vi "Encode Payload Data from Channels.vi"(6 "Offset":i32, 8 "error in":errorcluster, 9 "Parameters":T2(array[cluster]) {"encoding" items=["BNR", "BCD", "Discrete", "Signed_32", "Signed_64", "Float_32", "Float_64", "Opaque"]}, 10 "Data in":u8[](array[numeric]), 11 "Values in":dbl[](array[numeric])) -> (0 "error out":errorcluster, 2 "Data out":u8[](array[numeric]), 4 "Number of Parameters":i32)   [LabVIEW 2020]
uses:
  Encoding (Arinc664).ctl
  b24d3698-aaae-4200-bf93-4b6af5480478.vi
  5b1080be-549e-4688-aad8-fb955257d8ef.vi
  2afa5e5b-ae47-4ac6-b34f-e51087edfaba.vi
  1eaed3cb-9180-4944-bca4-c812fd7aad88.vi
  f46899e6-f3c2-4da0-acc2-ed34a334556c.vi
  7b487445-4b60-493e-9c15-0f5b7677c2b1.vi
  7e7e8f0d-6015-4215-b4f4-37ecf7ce16f3.vi
  b24d3698-aaae-4200-bf93-4b6af5480478.vi/9377bb8f-44b5-4a8f-87f1-966fd5a9edcc.vi
  b24d3698-aaae-4200-bf93-4b6af5480478.vi/e95d9d1f-307c-44d6-9f26-c3f519a4990d.vi
  b24d3698-aaae-4200-bf93-4b6af5480478.vi/0c23f515-4369-4514-bc3d-4444e6b437b2.vi
  5b1080be-549e-4688-aad8-fb955257d8ef.vi/136dcdcb-2dd3-4a4d-a796-a8f7a3f8e1ac.vi
  5b1080be-549e-4688-aad8-fb955257d8ef.vi/a54b505c-1216-4ef4-8378-3ceda9d188df.vi
  <vilib>/NI/NI VeriStand Encoding and Decoding/Get Bits Per Digit from Base.vi
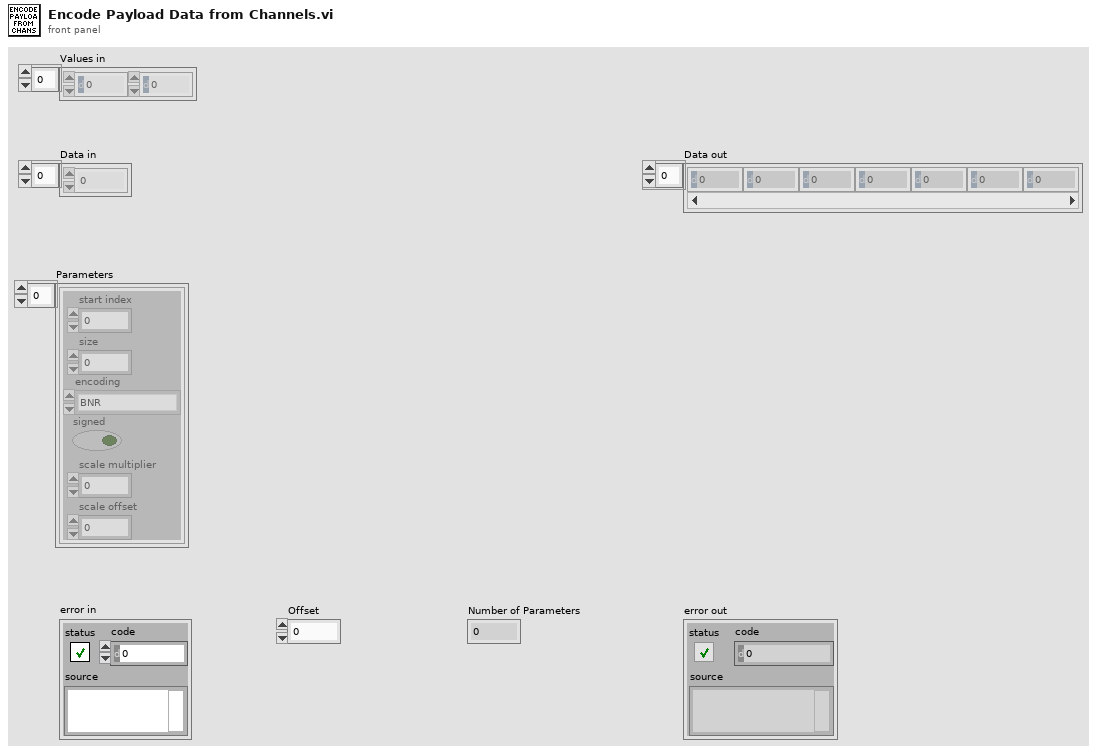
[diagram p1: front panel]
types:
  T1 = typedef "Encoding (Arinc664).ctl" = u16
  T2 = cluster{"start index":i32, "size":i32, "encoding":T1, "signed":bool, "scale multiplier":dbl, "scale offset":dbl}[]
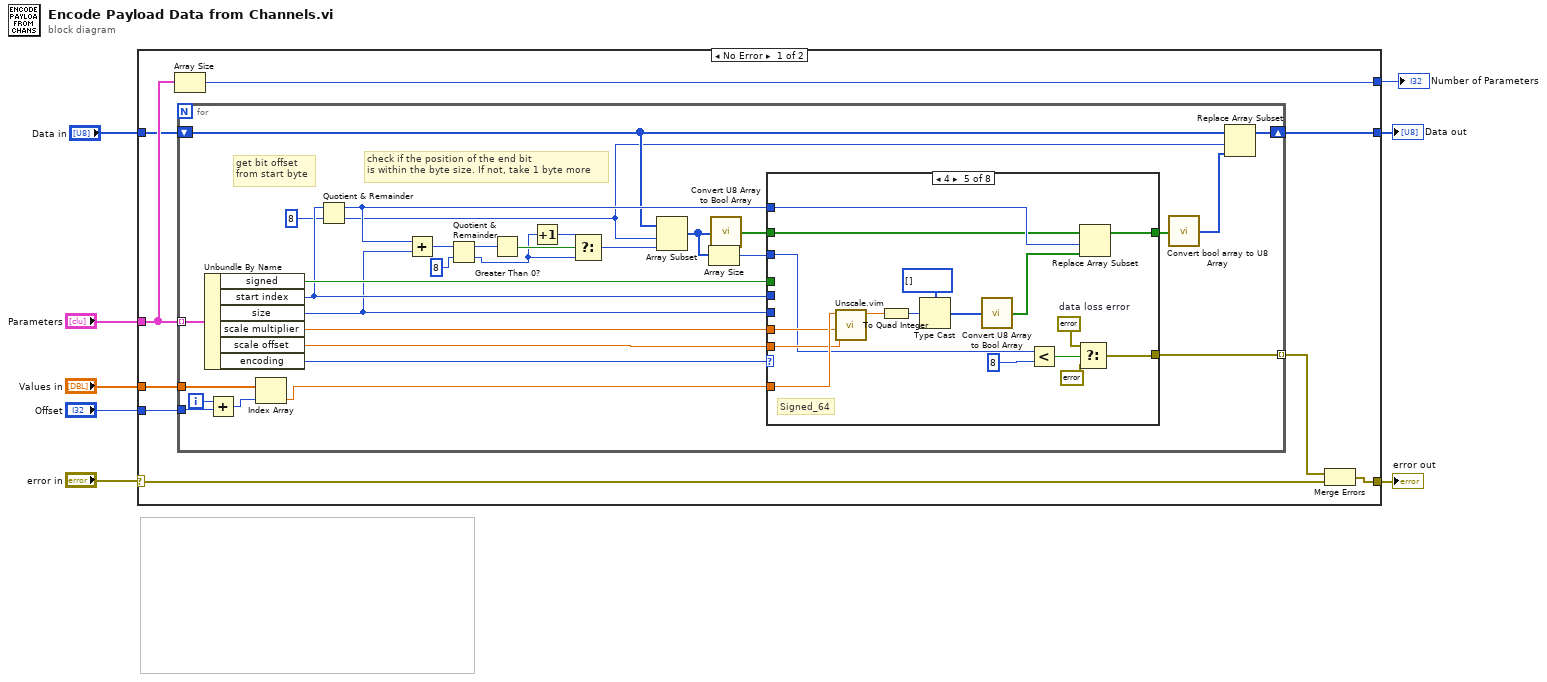
[diagram p0: block diagram]
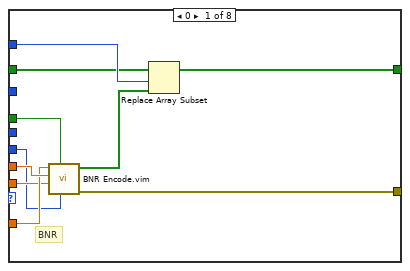
[diagram p2: hidden frame]
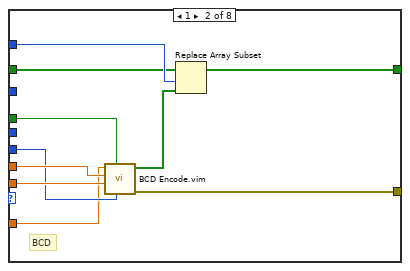
[diagram p3: hidden frame]
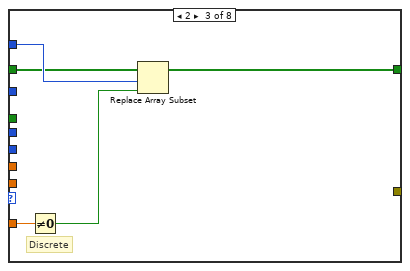
[diagram p4: hidden frame]
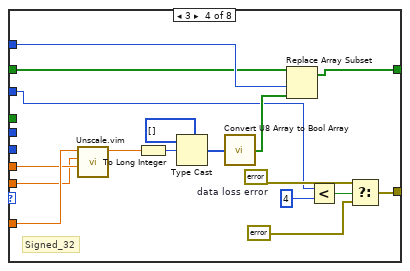
[diagram p5: hidden frame]
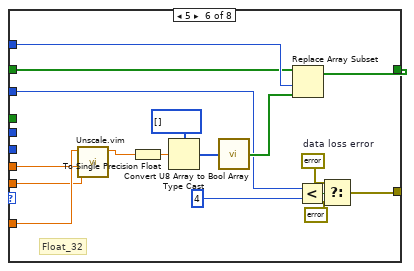
[diagram p6: hidden frame]
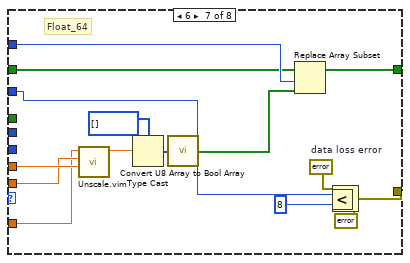
[diagram p7: hidden frame]
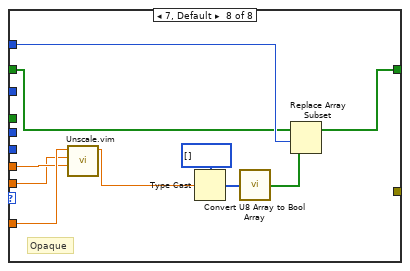
[diagram p8: hidden frame]
diagram:
  n1 = case shown="No Error" "error in" {
    selector: "error in" -> [w13 w151]
    tunnel: "Values in" -> [w17 _]
    tunnel: [w16 w150] -> w7
    tunnel: [w14 w151] -> w5
    tunnel: "Offset" -> [w12 _]
    tunnel: [w11 _] -> w3
    tunnel: "Parameters" -> [w10 _]
    tunnel: "Data in" -> [w9 w150]
    frame No Error {
      n2 = Array Size(array=w10) -> (size(s)=w11:i32)
      n3 = for {
        tunnel: w17 -> [w46]
        tunnel: w10 -> [w47] mode=indexing
        shift-right: [w24] -> w16
        shift-left: w9 -> [w25]
        tunnel: [w45] -> w15 mode=indexing
        tunnel: w12 -> [w43]
        i -> [w44]
        # "check if the position of the end bit \nis within the byte size. If not, take 1 byte more"
        # "get bit offset\nfrom start byte"
        n4 = Unbundle By Name(w47) -> ("signed"=w37:bool, "start index"=w36:i32, "size"=w33:i32, "scale multiplier"=w39:dbl, "scale offset"=w38:dbl, "encoding"=w40:T1)
        n5 = Add(x=w44, y=w43) -> (x+y=w42:i32)
        n6 = Index Array(array=w46, index=w42) -> (element=w41:dbl)
        n7 = Quotient & Remainder(x=w36, y=8) -> (x-y*floor(x/y)=w34:i32, floor(x/y)=w21:i32)
        n8 = Add(x=w34, y=w33) -> (x+y=w32:i32)
        n9 = Quotient & Remainder(x=w32, y=8) -> (x-y*floor(x/y)=w30:i32, floor(x/y)=w28:i32)
        n10 = Greater Than 0?(x=w30) -> (x > 0?=w29:bool)
        n11 = Increment(x=w28) -> (x+1=w27:i32)
        n12 = Select(t=w27, s=w29, f=w28) -> (s? t:f=w20:i32)
        n13 = Array Subset(array=w25, index=w21, length=w20) -> (w18:u8[])
        n14 = Array Size(array=w18) -> (size(s)=w19:i32)
        n15 = call "Convert U8 Array to Bool Array.vi"("U8 array in"=w18) -> ("Boolean array out"=w26:bool[])  [unwired: 14 in]
        n16 = case shown="4" w40 {
          tunnel: w37 -> [w57 w67 _ _ _ _ _ _]
          tunnel: w39 -> [w56 w66 _ w87 w104 w121 w138 w147]
          tunnel: w38 -> [w54 w65 _ w86 w103 w120 w137 w146]
          tunnel: w36 -> [_ _ _ _ _ _ _ _]
          tunnel: w33 -> [w53 w64 _ _ _ _ _ _]
          tunnel: w41 -> [w55 w62 w71 w88 w105 w122 w128 w148]
          tunnel: w34 -> [w52 w60 w72 w89 w106 w123 w139 w149]
          tunnel: [w50 w63 _ w80 w97 w114 w132 _] -> w45
          tunnel: w26 -> [w49 w59 w69 w75 w91 w108 w126 w141]
          tunnel: [w48 w58 w68 w74 w92 w109 w124 w140] -> w23
          tunnel: w19 -> [_ _ _ w73 w90 w107 w125 _]
          frame 0 {
            # "BNR"
            n17 = call "BNR Encode.vim"("data size (bits)"=w53, "signed"=w57, "scale offset"=w54, "scale multiplier"=w56, "value"=w55) -> ("error out"=w50:errorcluster, "BNR encoded value"=w51:bool[])  [unwired: 5 in]
            n18 = Replace Array Subset(array=w49, new element=w51, index=w52) -> (w48:bool[])
          }
          frame 1 {
            # "BCD"
            n19 = call "BCD Encode.vim"("data size (bits)"=w64, "signed"=w67, "scale offset"=w65, "scale multiplier"=w66, "value"=w62) -> ("error out"=w63:errorcluster, "BCD encoded value"=w61:bool[])  [unwired: 4 in, 1 out]
            n20 = Replace Array Subset(array=w59, new element=w61, index=w60) -> (w58:bool[])
          }
          frame 2 {
            # "Discrete"
            n21 = Not Equal To 0?(x=w71) -> (x != 0?=w70:bool)
            n22 = Replace Array Subset(array=w69, new element=w70, index=w72) -> (w68:bool[])
          }
          frame 3 {
            w81 = errorcluster {"status"=TRUE, "code"=-732301, "source"="data loss during encoding"}  # data loss error
            # "Signed_32"
            n23 = call "Unscale.vim"("scale multiplier"=w87, "scale offset"=w86, "value"=w88) -> ("unscaled value"=w85:dbl)  [unwired: 8 in]
            n24 = To Long Integer(number=w85) -> (32bit integer=w76:i32)
            n25 = Type Cast(type=u8[] [] ("subarray"), x=w76) -> (*(type *) &x=w83:u8[])
            n26 = call "Convert U8 Array to Bool Array.vi"("U8 array in"=w83) -> ("Boolean array out"=w82:bool[])  [unwired: 14 in]
            n27 = Replace Array Subset(array=w75, new element=w82, index=w89) -> (w74:bool[])
            n28 = Less?(x=w73, y=4) -> (x < y?=w78:bool)
            n29 = Select(t=w81, s=w78, f=errorcluster {"status"=FALSE, "code"=0, "source"=""}) -> (s? t:f=w80:errorcluster)
          }
          frame 4 {
            w98 = errorcluster {"status"=TRUE, "code"=-732301, "source"="data loss during encoding"}  # data loss error
            # "Signed_64"
            n30 = call "Unscale.vim"("scale multiplier"=w104, "scale offset"=w103, "value"=w105) -> ("unscaled value"=w102:dbl)  [unwired: 8 in]
            n31 = To Quad Integer(1:w102) -> (0:w93:i64)
            n32 = Type Cast(type=u8[] [] ("subarray"), x=w93) -> (*(type *) &x=w100:u8[])
            n33 = call "Convert U8 Array to Bool Array.vi"("U8 array in"=w100) -> ("Boolean array out"=w99:bool[])  [unwired: 14 in]
            n34 = Less?(x=w90, y=8) -> (x < y?=w95:bool)
            n35 = Select(t=w98, s=w95, f=errorcluster {"status"=FALSE, "code"=0, "source"=""}) -> (s? t:f=w97:errorcluster)
            n36 = Replace Array Subset(array=w91, new element=w99, index=w106) -> (w92:bool[])
          }
          frame 5 {
            w115 = errorcluster {"status"=TRUE, "code"=-732301, "source"="data loss during encoding"}  # data loss error
            # "Float_32"
            n37 = call "Unscale.vim"("scale multiplier"=w121, "scale offset"=w120, "value"=w122) -> ("unscaled value"=w119:dbl)  [unwired: 8 in]
            n38 = To Single Precision Float(number=w119) -> (single precision float=w110:sgl)
            n39 = Type Cast(type=u8[] [] ("subarray"), x=w110) -> (*(type *) &x=w117:u8[])
            n40 = call "Convert U8 Array to Bool Array.vi"("U8 array in"=w117) -> ("Boolean array out"=w116:bool[])  [unwired: 14 in]
            n41 = Replace Array Subset(array=w108, new element=w116, index=w123) -> (w109:bool[])
            n42 = Less?(x=w107, y=4) -> (x < y?=w112:bool)
            n43 = Select(t=w115, s=w112, f=errorcluster {"status"=FALSE, "code"=0, "source"=""}) -> (s? t:f=w114:errorcluster)
          }
          frame 6 {
            w133 = errorcluster {"status"=TRUE, "code"=-732301, "source"="data loss during encoding"}  # data loss error
            # "Float_64"
            n44 = call "Unscale.vim"("scale multiplier"=w138, "scale offset"=w137, "value"=w128) -> ("unscaled value"=w127:dbl)  [unwired: 8 in]
            n45 = Type Cast(type=u8[] [] ("subarray"), x=w127) -> (*(type *) &x=w135:u8[])
            n46 = call "Convert U8 Array to Bool Array.vi"("U8 array in"=w135) -> ("Boolean array out"=w134:bool[])  [unwired: 14 in]
            n47 = Replace Array Subset(array=w126, new element=w134, index=w139) -> (w124:bool[])
            n48 = Less?(x=w125, y=8) -> (x < y?=w130:bool)
            n49 = Select(t=w133, s=w130, f=errorcluster {"status"=FALSE, "code"=0, "source"=""}) -> (s? t:f=w132:errorcluster)
          }
          frame 7, Default {
            # "Opaque"
            n50 = call "Unscale.vim"("scale multiplier"=w147, "scale offset"=w146, "value"=w148) -> ("unscaled value"=w145:dbl)  [unwired: 8 in]
            n51 = Type Cast(type=u8[] [] ("subarray"), x=w145) -> (*(type *) &x=w143:u8[])
            n52 = call "Convert U8 Array to Bool Array.vi"("U8 array in"=w143) -> ("Boolean array out"=w142:bool[])  [unwired: 14 in]
            n53 = Replace Array Subset(array=w141, new element=w142, index=w149) -> (w140:bool[])
          }
        }
        n54 = call "Convert bool array to U8 Array.vi"("Boolean array"=w23) -> ("Array"=w22:u8[])  [unwired: 14 in]
        n55 = Replace Array Subset(array=w25, new element=w22, index=w21) -> (w24:u8[])
      }
      n56 = Merge Errors(w15, w13) -> (w14:errorcluster)
    }
    frame Error {
    }
  }
  "Data out" <- w7
  "error out" <- w5
  "Number of Parameters" <- w3
